vi "Add Client to Service.vi"(8 "error in (no error)":errorcluster, 9 "Client ID":string, 10 "WebSocket Connection in":refnum<k5>, 11 "WebSocket Server in":refnum<class "WebSocket Server.lvclass">) -> (0 "error out":errorcluster, 3 "WebSocket Server out":refnum<class "WebSocket Server.lvclass">)   [LabVIEW 2016, in "WebSocket Actor.lvlib" / "WebSocket Server.lvclass"]
uses:
  WebSocket Server.lvclass
  WebSocket Server.lvclass/WebSocket Server.ctl
  Handshake Response Action.ctl
  Http Response Codes.ctl
  <vilib>/GPower/Error/Library/Filter/FilterSingle.vi
  <vilib>/GPower/Error/Library/SplitAppended.vi
  <vilib>/GPower/Error/Library/SubVIs/ExplanationToError.vi
  <vilib>/dlg_ctls.llb/Space Constant.vi
  <vilib>/Utility/error.llb/Trim Whitespace.vi
  <vilib>/Utility/error.llb/Error Code Database.vi
  <vilib>/GPower/Error/Library/Append/AppendSingle.vi
  <vilib>/MediaMongrels Ltd/WebSockets/WebSockets/WebSockets.lvlib
  <vilib>/GPower/Error/GPError.lvlib
  WebSocket Service Actor Messages/Add Client Msg/Add Client Msg.lvclass
panel:
  out "Request URI":string
  out "HTTP Headers":variant
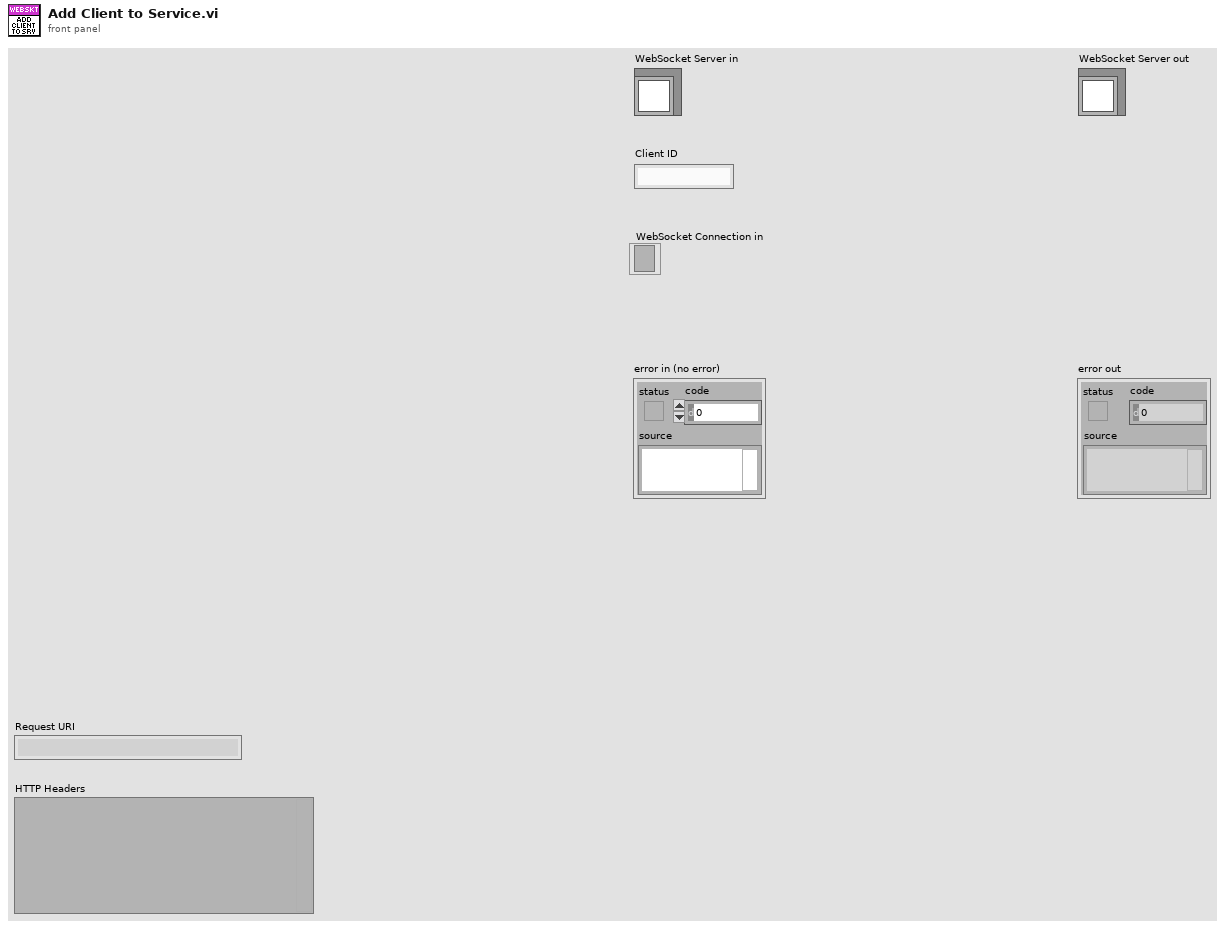
[diagram p1: front panel]
types:
  T1 = typedef "WebSocket Actor.lvlib/WebSocket Server.lvclass/Handshake Response Action.ctl" = enum16{"None", "Service Not Defined"}
  T2 = typedef "WebSocket Actor.lvlib/WebSocket Server.lvclass/Http Response Codes.ctl" = u16
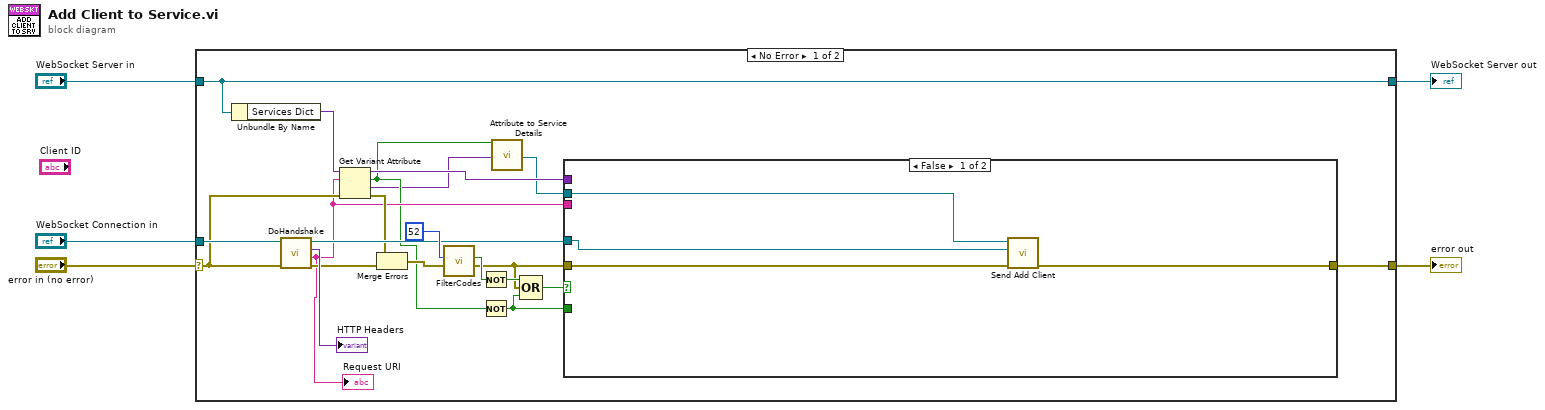
[diagram p0: block diagram]
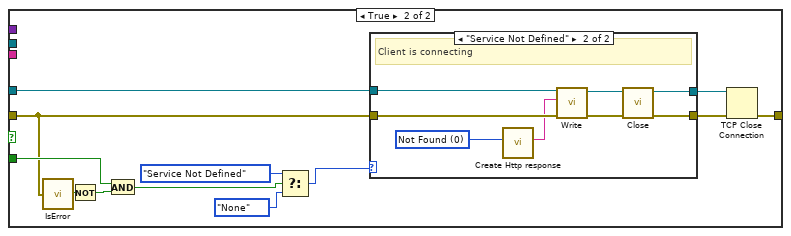
[diagram p2: hidden frame]
diagram:
  n1 = case shown="No Error" "error in (no error)" {
    selector: "error in (no error)" -> [w16 w54]
    tunnel: [w6 w54] -> w4
    tunnel: [w18 w53] -> w2
    tunnel: "WebSocket Server in" -> [w18 w53]
    tunnel: "WebSocket Connection in" -> [w19 _]
    frame No Error {
      n2 = Unbundle By Name(w18) -> ("Services Dict"=w17:variant)
      n3 = call <vilib>:"DoHandshake.vi"("error in (no error)"=w16, "WebSocket Connection in"=w19) -> ("error out"=w15:errorcluster, "Request URI"=w10:string, "Headers Out"=→"HTTP Headers":variant, "WebSocket Connection out"=w21:refnum<k5>)  [unwired: 6 in]
      "Request URI" <- w10
      n4 = Get Variant Attribute(Variant=w17, name=w10, error in=w16) -> (duplicate Variant=w14:variant, found=w9:bool, value=w8:variant, error out=w12:errorcluster)  [unwired: 1 in]
      n5 = Merge Errors(w12, w15) -> (w13:errorcluster)
      n6 = call-poly <vilib>:"FilterCodes.vi"("Error in"=w13, "Code to filter"=52) -> ("Error out"=w20:errorcluster, "Code filtered?"=w24:bool)  [unwired: 8 in]
      n7 = Not(x=w24) -> (.not. x?=w23:bool)
      n8 = Not(x=w9) -> (.not. x?=w11:bool)
      n9 = call "Attribute to Service Details.vi"("Attibute Found"=w9, "Attribute"=w8) -> ("Service Enqueuer"=w7:refnum<class "Message Enqueuer.lvclass">)  [unwired: 17 in]
      n10 = Compound Arithmetic op=OR(w23, w20, w11) -> (w22:bool)
      n11 = case shown="False" w22 {
        tunnel: w21 -> [w27 w40]
        tunnel: w20 -> [w30 w34]
        tunnel: [w29 w42] -> w6
        tunnel: w14 -> [_ _]
        tunnel: w11 -> [_ w36]
        tunnel: w10 -> [_ _]
        tunnel: w7 -> [w28 _]
        frame False {
          n12 = call "Send Add Client.vi"("error in (no error)"=w30, "WebSocket Connection"=w27, "Message Enqueuer in"=w28) -> ("error out"=w29:errorcluster)  [unwired: 7 in, 1 out]
        }
        frame True {
          n13 = call <vilib>:"IsError.vi"("Error in"=w34) -> ("Error?"=w33:bool)  [unwired: 4 in]
          n14 = Not(x=w33) -> (.not. x?=w31:bool)
          n15 = And(x=w36, y=w31) -> (x .and. y?=w32:bool)
          n16 = Select(t=Handshake_Response_Action."Service Not Defined" ("Response Action"), s=w32, f=Handshake_Response_Action."None") -> (s? t:f=w37:T1)
          n17 = case shown="\"Service Not Defined\"" w37 {
            tunnel: w34 -> [w44 w52]
            tunnel: [w44 w50] -> w41
            tunnel: w40 -> [w43 w47]
            tunnel: [w43 w45] -> w39
            frame "None", Default {
            }
            frame "Service Not Defined" {
              w49 = T2 0 items=["Forbidden"=403, "Not Found"=0, "Upgrade Required"=426] ("Http Response Codes")
              # "Client is connecting"
              n18 = call "Create Http response.vi"("Http Response Codes"=w49) -> ("Http Response"=w48:string)  [unwired: 10 in]
              n19 = call <vilib>:"Write.vi"("error in (no error)"=w52, "Data"=w48, "WebSocket Connection in"=w47) -> ("error out"=w51:errorcluster, "WebSocket Connection out"=w46:refnum<k5>)  [unwired: 7 in]
              n20 = call <vilib>:"Close.vi"("error in (no error)"=w51, "WebSocket Connection in"=w46) -> ("error out"=w50:errorcluster, "WebSocket Connection in"=w45:refnum<k5>)  [unwired: 8 in]
            }
          }
          n21 = TCP Close Connection(connection ID=w39, error in (no error)=w41) -> (error out=w42:errorcluster)  [unwired: 1 in, 1 out]
        }
      }
    }
    frame Error {
    }
  }
  "error out" <- w4
  "WebSocket Server out" <- w2
